vi "SVT Weighting Filter (frequency).vi"   [LabVIEW 2017, in "SoundVib_ABCWeighting.lvlib"]
doc: "Applies the selected weighting to the <B>spectrum</B> or <B>spectra</B> in the frequency domain. This VI operates on Power, PSD, COP, FFT [Mag], FFT [Re], and FFT [Imag] spectra. Wire data to the <B>spectrum</B> input to determine the polymorphic instance to use or manually select the instance."
uses:
  <vilib>/addons/Sound and Vibration/svt_Weighting/SoundVib_ABCWeighting.lvlib
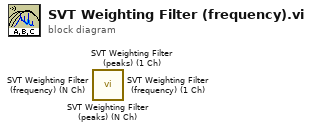
[diagram p0: block diagram]
diagram:
  n1 = call <vilib>:"SVT Weighting Filter (peaks) (N Ch).vi"() -> ()  [unwired: 16 in, 4 out]
  n2 = call <vilib>:"SVT Weighting Filter (peaks) (1 Ch).vi"() -> ()  [unwired: 16 in, 4 out]
  n3 = call <vilib>:"SVT Weighting Filter (frequency) (N Ch).vi"() -> ()  [unwired: 16 in, 4 out]
  n4 = call <vilib>:"SVT Weighting Filter (frequency) (1 Ch).vi"() -> ()  [unwired: 16 in, 4 out]
